vi "ExplorerTree Recursive FilesV2.vi"(4 "Folder to Exclude":string[](array[string]), 6 "Pattern":string, 8 "error in (no error)":errorcluster, 9 "Continue Recursing on Error? (F)":bool, 10 "FilePaths to Exclude":path[](array[path]), 11 "Folder Path":path) -> (0 "error out":errorcluster, 1 "Folder Indexes":i32[](array[numeric]), 2 "Folders and Files":path[](array[path]), 3 "dup Folder Path":path)   [LabVIEW 2023]
doc: "List the content of a folder sorted by directories first. The <b>Folder Indexes</b> contain the index locations of the directories in the <b>Folders and Files</b> paths array. All other indexes are files.\n\nCreated By: Ryan Pacini"
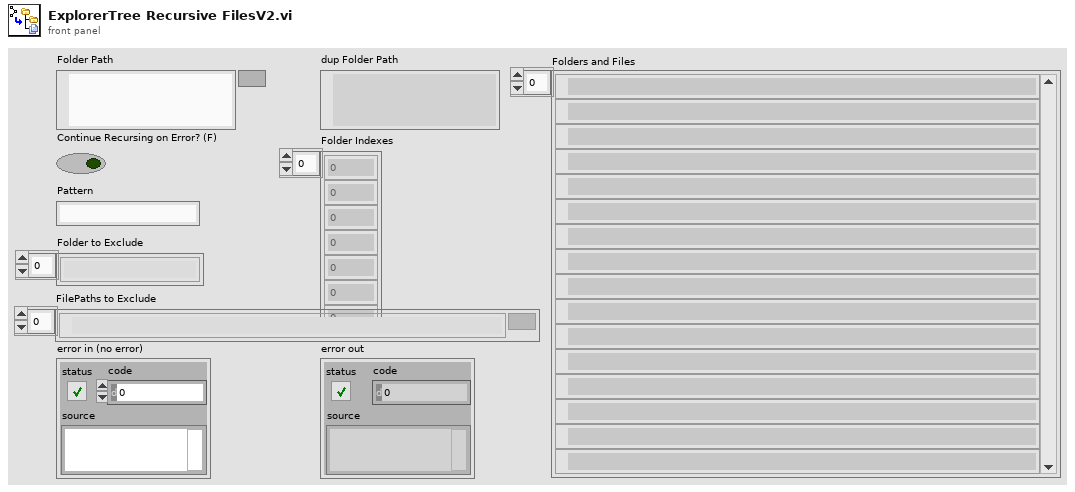
[diagram p1: front panel]
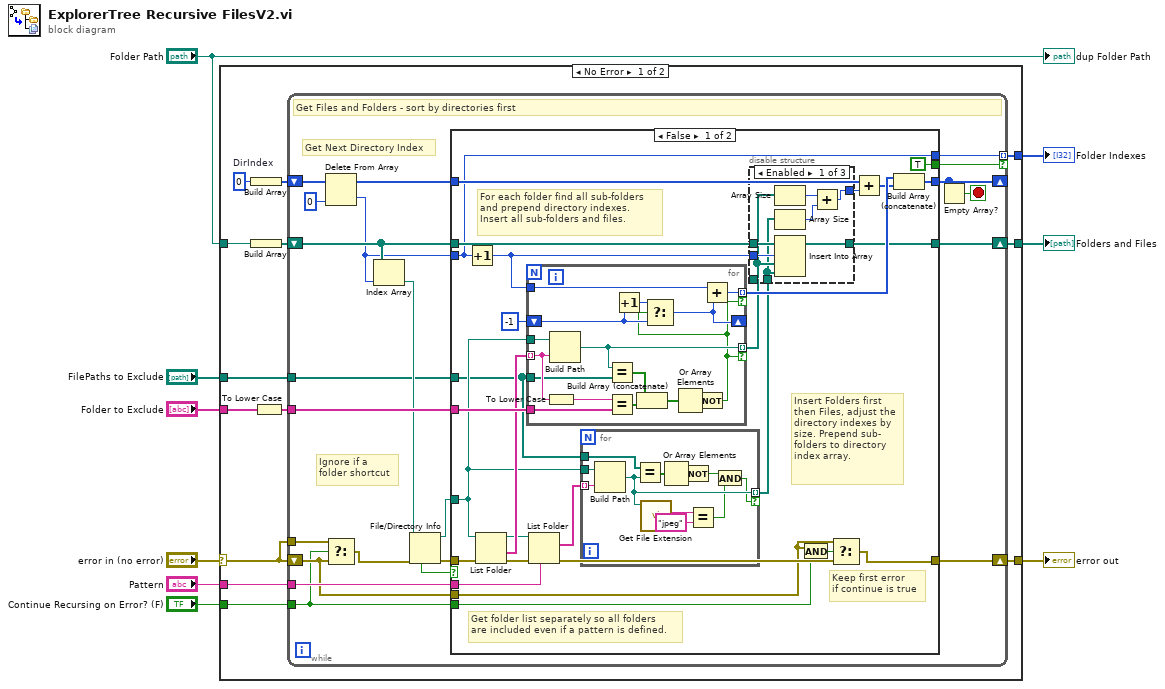
[diagram p0: block diagram]
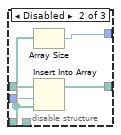
[diagram p2: hidden frame]
diagram:
  n1 = case shown="No Error" "error in (no error)" {
    selector: "error in (no error)" -> [w13 w115]
    tunnel: "Folder to Exclude" -> [w22 _]
    tunnel: [w20 w115] -> w8
    tunnel: "Pattern" -> [w19 _]
    tunnel: [w15 _] -> w6
    tunnel: "Folder Path" -> [w14 _]
    tunnel: "Continue Recursing on Error? (F)" -> [w12 _]
    tunnel: [w11 _] -> w2
    tunnel: "FilePaths to Exclude" -> [w10 _]
    frame No Error {
      w17 = 0  # DirIndex
      n2 = Build Array(w17) -> (w16:i32[])
      n3 = Build Array(w14) -> (w18:path[])
      n4 = To Lower Case(string=w22) -> (all lower case string=w21:string[])
      n5 = while {
        tunnel: w21 -> [w40]
        tunnel: w19 -> [w39]
        shift-right: [w38] -> w15
        shift-left: w18 -> [w37]
        shift-right: [w31] -> _
        shift-left: w16 -> [w35]
        shift-right: [w26] -> w20
        shift-left: w13 -> [w28]
        tunnel: w13 -> [w29]
        tunnel: w12 -> [w27]
        tunnel: [w25] -> w11 mode=indexing if=w24
        tunnel: w10 -> [w23]
        stop <- w41 stop-if-true
        # "Ignore if a\nfolder shortcut"
        # "Get Next Directory Index"
        # "Get Files and Folders - sort by directories first"
        n6 = Delete From Array(array=w35, index=0) -> (deleted portion=w34:i32, array with subset deleted=w32:i32[])  [unwired: 1 in]
        n7 = Select(t=w29, s=w27, f=w28) -> (s? t:f=w30:errorcluster)
        n8 = Index Array(array=w37, index=w34) -> (element=w36:path)
        n9 = File/Directory Info(path=w36, error in=w30) -> (path out=w43:path, error out=w44:errorcluster, shortcut=w42:bool)  [unwired: 4 out]
        n10 = case shown="False" w42 {
          tunnel: w44 -> [w71 w114]
          tunnel: w43 -> [w64 _]
          tunnel: [w55 w114] -> w26
          tunnel: w40 -> [w70 _]
          tunnel: [w48 w113] -> w38
          tunnel: w39 -> [w65 _]
          tunnel: w37 -> [w63 w113]
          tunnel: w34 -> [w51 _]
          tunnel: w32 -> [w58 w112]
          tunnel: [w60 w112] -> w31
          tunnel: w28 -> [w53 _]
          tunnel: w27 -> [w54 _]
          tunnel: [w51 _] -> w25
          tunnel: [TRUE _] -> w24
          tunnel: w23 -> [w45 _]
          frame False {
            # "Insert Folders first\nthen Files, adjust the\ndirectory indexes by\nsize. Prepend sub-\nfolders to directory\nindex array."
            # "Keep first error\nif continue is true"
            # "Get folder list separately so all folders \nare included even if a pattern is defined."
            # "For each folder find all sub-folders\nand prepend directory indexes.\nInsert all sub-folders and files."
            n11 = Increment(x=w51) -> (x+1=w62:i32)
            n12 = List Folder(path=w64, error in=w71) -> (path out=w66:path, folder names=w69:string[], error out=w67:errorcluster)  [unwired: 2 in, 1 out]
            n13 = for {
              tunnel: w69 -> [w106] mode=indexing
              tunnel: w64 -> [w111]
              tunnel: w70 -> [w109]
              tunnel: [w100] -> w59 mode=indexing if=w98
              tunnel: w62 -> [w105]
              tunnel: [w104] -> w61 mode=indexing if=w98
              shift-right: [w101] -> _
              shift-left: -1 -> [w102]
              tunnel: w45 -> [w99]
              # "Exclude Folders"
              n14 = To Lower Case(string=w106) -> (all lower case string=w110:string)
              n15 = Build Path(base path=w111, name or relative path=w106) -> (appended path=w100:path)
              n16 = Equal?(x=w100, y=w99) -> (x = y?=w96:bool[])
              n17 = Equal?(x=w110, y=w109) -> (x = y?=w108:bool[])
              n18 = Increment(x=w102) -> (x+1=w103:i32)
              n19 = Build Array (concatenate)(w96, w108) -> (w97:bool[])
              n20 = Or Array Elements(Boolean array=w97) -> (logical OR=w107:bool)
              n21 = Not(x=w107) -> (.not. x?=w98:bool)
              n22 = Select(t=w103, s=w98, f=w102) -> (s? t:f=w101:i32)
              n23 = Add(x=w105, y=w101) -> (x+y=w104:i32)
            }
            n24 = List Folder(path=w66, pattern=w65, error in=w67) -> (filenames=w68:string[], error out=w56:errorcluster)  [unwired: 1 in, 2 out]
            n25 = for {
              tunnel: w64 -> [w95]
              tunnel: w68 -> [w94] mode=indexing
              tunnel: [w90] -> w47 mode=indexing if=w86
              tunnel: w45 -> [w93]
              n26 = Build Path(base path=w95, name or relative path=w94) -> (appended path=w90:path)
              n27 = Equal?(x=w93, y=w90) -> (x = y?=w91:bool[])
              n28 = call <vilib>:"Get File Extension.vi"("file"=w90) -> ("lowercase file extension"=w88:string)  [unwired: 6 in, 4 out]
              n29 = Or Array Elements(Boolean array=w91) -> (logical OR=w92:bool)
              n30 = Not(x=w92) -> (.not. x?=w89:bool)
              n31 = Equal?(x=w88, y="jpeg") -> (x = y?=w87:bool)
              n32 = And(x=w89, y=w87) -> (x .and. y?=w86:bool)
            }
            n33 = disable-structure shown="Enabled" {
              disable-tunnel: w63 -> [w79 w84 _]
              disable-tunnel: w62 -> [w78 w83 _]
              disable-tunnel: w59 -> [w77 w82 _]
              disable-tunnel: [w75 w81 _] -> w48
              disable-tunnel: w47 -> [w74 _ _]
              disable-tunnel: [w73 w80 _] -> w46
              frame Enabled {
                n34 = Array Size(array=w77) -> (size(s)=w76:i32)
                n35 = Array Size(array=w74) -> (size(s)=w72:i32)
                n36 = Insert Into Array(array=w79, index=w78, new element #1=w77, new element #2=w74) -> (w75:path[])
                n37 = Add(x=w76, y=w72) -> (x+y=w73:i32)
              }
              frame Disabled {
                n38 = Array Size(array=w82) -> (size(s)=w80:i32)
                n39 = Insert Into Array(array=w84, index=w83, new element=w82) -> (w81:path[])
              }
              frame Disabled {
              }
            }
            n40 = And(x=w53, y=w54) -> (x .and. y?=w52:bool)
            n41 = Select(t=w53, s=w52, f=w56) -> (s? t:f=w55:errorcluster)
            n42 = Add(x=w58, y=w46) -> (x+y=w57:i32[])
            n43 = Build Array (concatenate)(w61, w57) -> (w60:i32[])
          }
          frame True {
            # "Directory is a shortcut, do nothing"
          }
        }
        n44 = Empty Array?(array=w31) -> (empty?=w41:bool)
      }
    }
    frame Error {
    }
  }
  "error out" <- w8
  "Folders and Files" <- w6
  "Folder Indexes" <- w2
  "dup Folder Path" <- "Folder Path"
